vi "stageToCam.vi"(6 "error in (no error)":errorcluster, 8 "center location":dbl[](array[numeric]), 9 "transform cluster + actuator":T1, 10 "current positions":T2, 11 "cam location (px)":dbl[](array[numeric])) -> (3 "stage location (steps)":dbl[](array[numeric]), 4 "error out":errorcluster)   [LabVIEW 2015]
uses:
  pipette cleaning/pressure box/cleaning_soft/controls/actuator_type.ctl
  pipette cleaning/pressure box/cleaning_soft/controls/actuator_cluster.ctl
  transform_properties_actuators.ctl
  controls/transform_cluster_actuator.ctl
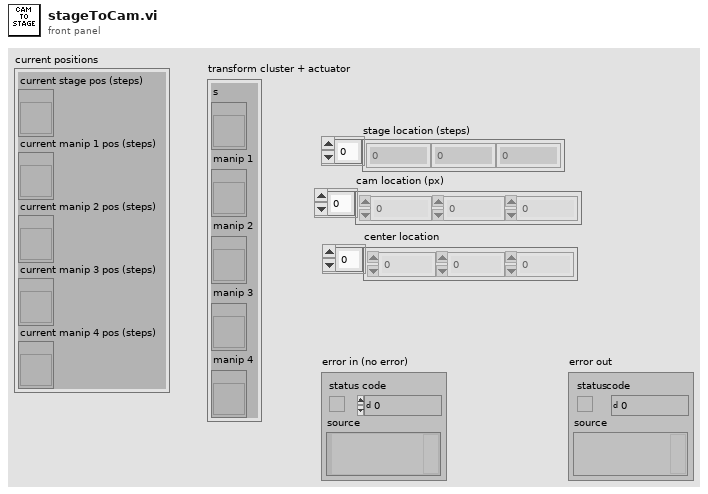
[diagram p1: front panel]
types:
  T1 = typedef "transform_cluster_actuator.ctl" = cluster{"s":refnum<vi>, "manip 1":refnum<vi>, "manip 2":refnum<vi>, "manip 3":refnum<vi>, "manip 4":refnum<vi>}
  T2 = cluster{"current stage pos (steps)":refnum<vi>, "current manip 1 pos (steps)":refnum<vi>, "current manip 2 pos (steps)":refnum<vi>, "current manip 3 pos (steps)":refnum<vi>, "current manip 4 pos (steps)":refnum<vi>}
  T3 = typedef "transform_properties_actuators.ctl" = cluster{"theta (deg)":dbl, "X sc factor (px/step)":dbl, "Y sc factor (px/step)":dbl, "zero loc (x,y,z)":dbl[], "flip y?":bool, "flip x?":bool, "gamma (deg)":dbl, "flip z?":bool, "Z sc factor (px/step)":dbl, "actuator":T4, "safe space (steps)":i32[]}
  T4 = typedef "actuator_cluster.ctl" = cluster{"Actuator COM":refnum<visa-resource-name>, "Actuator type":T5}
  T5 = typedef "actuator_type.ctl" = enum16{"Scientifica", "Sutter", "Demo", "Off"}
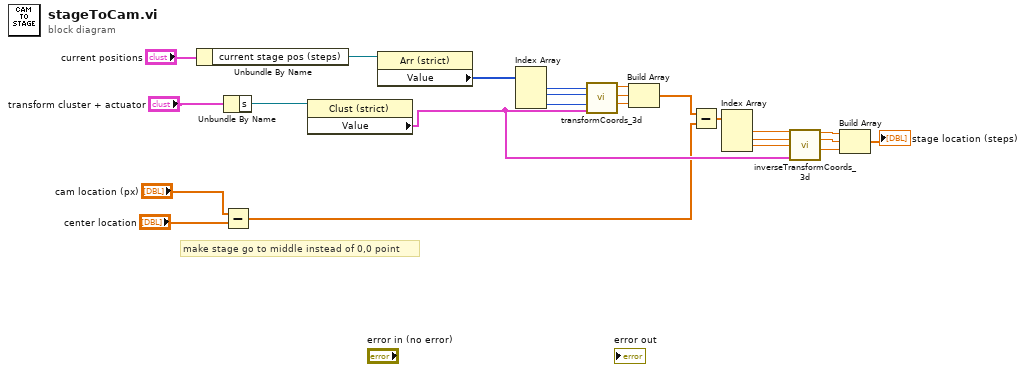
[diagram p0: block diagram]
diagram:
  # "make stage go to middle instead of 0,0 point"
  n1 = Unbundle By Name("current positions") -> ("current stage pos (steps)"=w23:refnum<vi>)
  n2 = Subtract(x="cam location (px)", y="center location") -> (x-y=w6:dbl[])
  n3 = Unbundle By Name("transform cluster + actuator") -> ("s"=w19:refnum<vi>)
  n4 = property class="Clust (strict)"(reference=w19) -> ("Value"=w12:T3)  [unwired: 1 in, 2 out]
  n5 = property class="Arr (strict)"(reference=w23) -> ("Value"=w22:i32[])  [unwired: 1 in, 2 out]
  n6 = Index Array(array=w22) -> (element #1=w21:i32, element #2=w20:i32, element #3=w4:i32)  [unwired: 3 in]
  n7 = call "transformCoords_3d.vi"("transform properties"=w12, "z"=w4, "y"=w20, "x"=w21) -> ("z out"=w3:dbl, "y out"=w17:dbl, "x out"=w18:dbl)  [unwired: 5 in]
  n8 = Build Array(w18, w17, w3) -> (w16:dbl[])
  n9 = Subtract(x=w16, y=w6) -> (x-y=w15:dbl[])
  n10 = Index Array(array=w15) -> (element #1=w14:dbl, element #2=w13:dbl, element #3=w2:dbl)  [unwired: 3 in]
  n11 = call "inverseTransformCoords_3d.vi"("x"=w14, "y"=w13, "z"=w2, "transform properties"=w12) -> ("x out"=w11:dbl, "y out"=w10:dbl, "z out"=w1:dbl)  [unwired: 9 in]
  n12 = Build Array(w11, w10, w1) -> (→"stage location (steps)":dbl[])
